vi "UpdateMotors.vi"(2 "Speed Fraction":dbl min=-1.0 max=1.0 step=0.01, 3 "Spin Fraction":dbl min=-1.0 max=1.0 step=0.001, 5 "Motor PWMs":T8) -> ()   [LabVIEW 2015]
uses:
  <vilib>/myRIO/Instrument Drivers/Onboard IO/PWM/typedefs/PWM Reference.ctl
  <vilib>/myRIO/Common/Instrument Driver Framework/Utilities/typedefs/myRIO Generic Hardware Reference.ctl
  <vilib>/myRIO/Common/Instrument Driver Framework/Utilities/typedefs/Hardware Version Enum.ctl
  <vilib>/myRIO/Common/Instrument Driver Framework/Utilities/typedefs/myRIO v1.0 Reference.ctl
  <vilib>/myRIO/Common/Instrument Driver Framework/Utilities/typedefs/Generic FPGA Reference.ctl
  <vilib>/myRIO/Common/Instrument Driver Framework/myRIO v1.0/PWM/typedefs/PWM Channels Enum.ctl
  <vilib>/myRIO/Instrument Drivers/Onboard IO/PWM/typedefs/PWM Configuration.ctl
  <vilib>/myRIO/Instrument Drivers/Onboard IO/PWM/vis/Set Duty Cycle and Frequency.vi
  <vilib>/Utility/error.llb/Error Cluster From Error Code.vi
  <vilib>/myRIO/Common/Instrument Driver Framework/myRIO v1.0/PWM/vis/myRIO v1.0 Write PWM.vi
  <vilib>/myRIO/Instrument Drivers/Onboard IO/PWM/PWM.lvlib
panel:
  out "Waveform Chart 2":dbl(graph)
  out "Waveform Chart":dbl(graph)
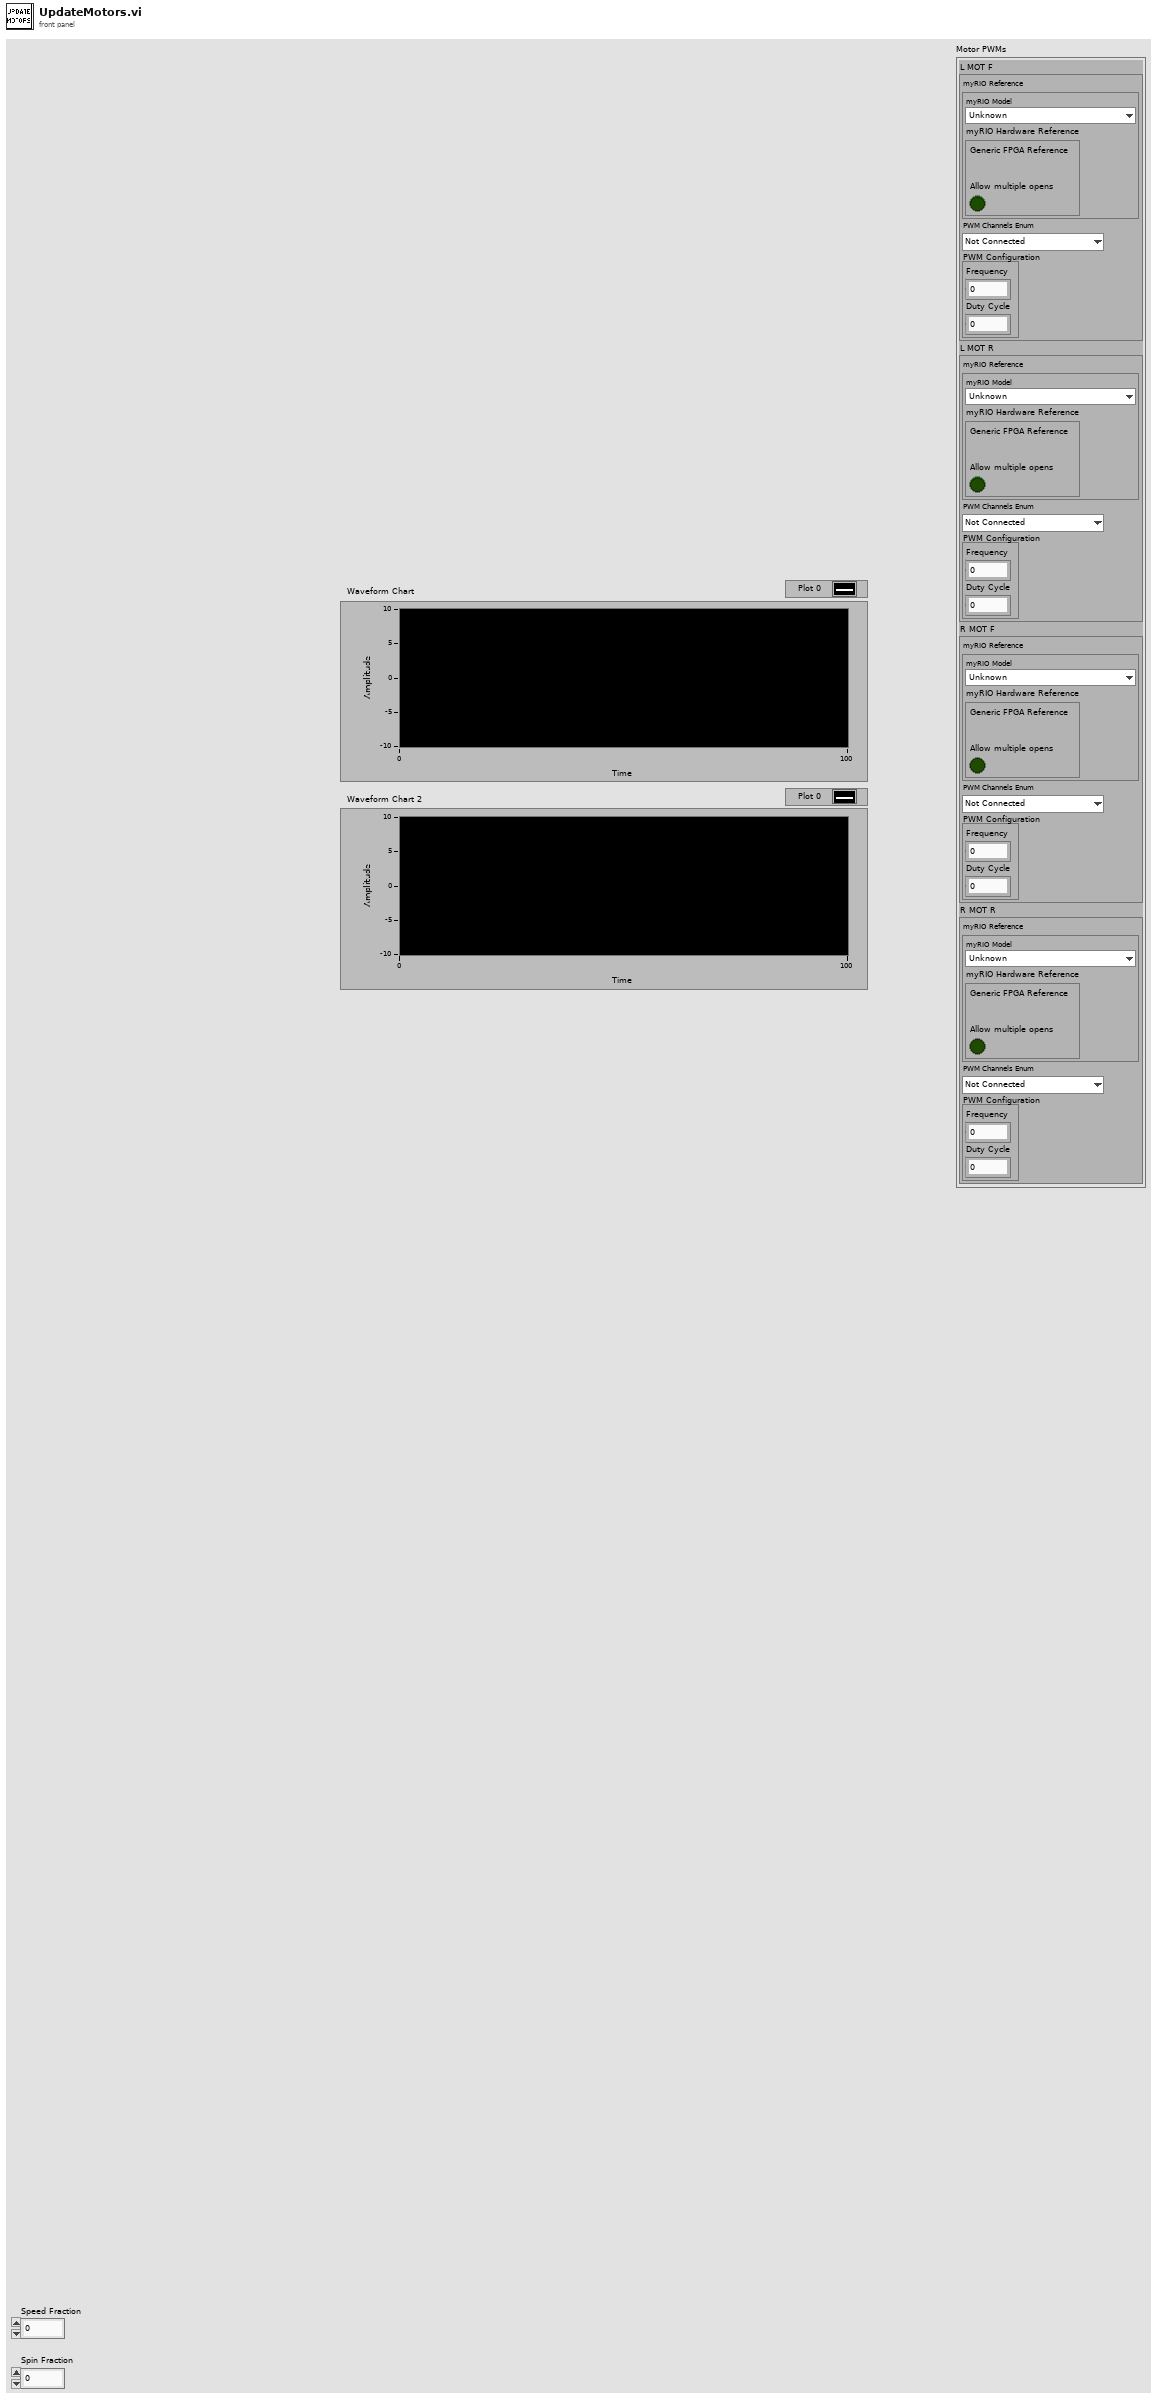
[diagram p1: front panel]
types:
  T1 = typedef "PWM.lvlib/PWM Reference.ctl" = cluster{"myRIO Reference":T2, "PWM Channels Enum":T6, "PWM Configuration":T7}
  T2 = typedef "myRIO Generic Hardware Reference.ctl" = cluster{"myRIO Model":T3, "myRIO Hardware Reference":T4}
  T3 = typedef "Hardware Version Enum.ctl" = enum16{"Unknown", "myRIO-1900", "myRIO-1950", "roboRIO"}
  T4 = typedef "myRIO v1.0 Reference.ctl" = cluster{"Generic FPGA Reference":T5, "Allow multiple opens":bool}
  T5 = typedef "Generic FPGA Reference.ctl" = refnum<k20>
  T6 = typedef "PWM Channels Enum.ctl" = enum16{"Not Connected", "C/PWM0", "C/PWM1", "A/PWM0", "A/PWM1", "A/PWM2", "B/PWM0", "B/PWM1", "B/PWM2", "PWM/PWM0", "PWM/PWM1", "PWM/PWM2", "PWM/PWM3", "PWM/PWM4", "PWM/PWM5", "PWM/PWM6", "PWM/PWM7", "PWM/PWM8", "PWM/PWM9"}
  T7 = typedef "PWM.lvlib/PWM Configuration.ctl" = cluster{"Frequency":dbl, "Duty Cycle":dbl}
  T8 = cluster{"L MOT F ":T1, "L MOT R":T1, "R MOT F":T1, "R MOT R":T1}
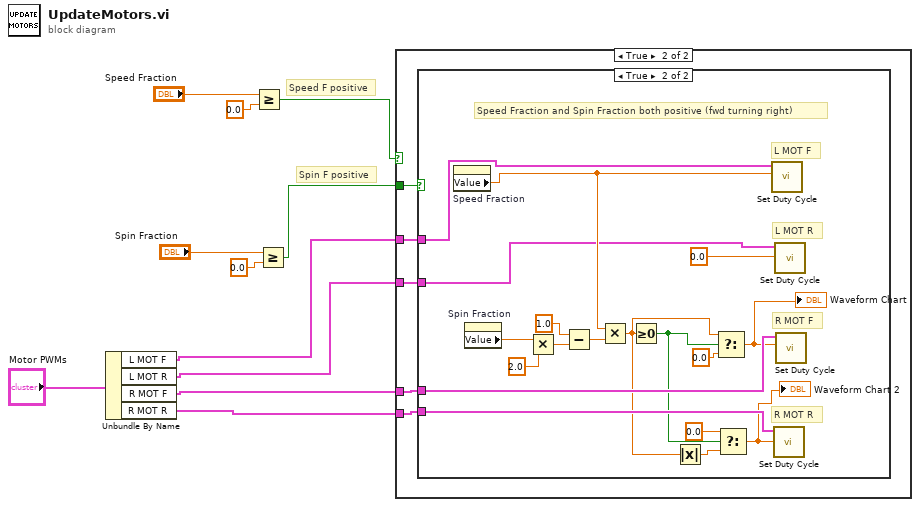
[diagram p0: block diagram]
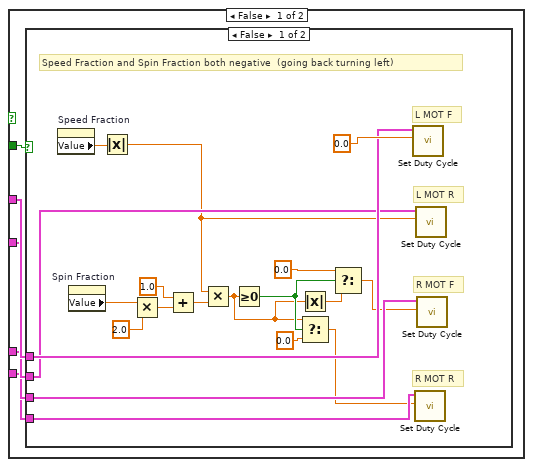
[diagram p2: hidden frame]
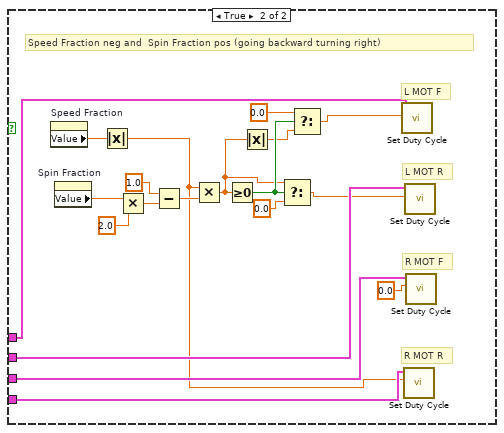
[diagram p3: hidden frame]
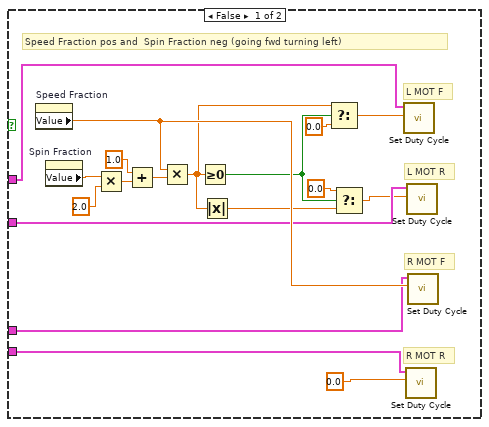
[diagram p4: hidden frame]
diagram:
  # "Spin F positive"
  # "Speed F positive"
  n1 = Unbundle By Name("Motor PWMs") -> ("L MOT F"=w5:T1, "L MOT R"=w4:T1, "R MOT F"=w3:T1, "R MOT R"=w2:T1)
  n2 = Greater Or Equal?(x="Speed Fraction", y=0.0) -> (x >= y?=w7:bool)
  n3 = Greater Or Equal?(x="Spin Fraction", y=0.0) -> (x >= y?=w6:bool)
  n4 = case shown="True" w7 {
    tunnel: w6 -> [w16 w59]
    tunnel: w5 -> [w15 w58]
    tunnel: w4 -> [w14 w57]
    tunnel: w3 -> [w13 w56]
    tunnel: w2 -> [w12 w55]
    frame False {
      n5 = case shown="False" w16 {
        tunnel: w15 -> [w29 w48]
        tunnel: w14 -> [w28 w47]
        tunnel: w13 -> [w27 w46]
        tunnel: w12 -> [w26 w45]
        frame False {
          # "Speed Fraction and Spin Fraction both negative  (going back turning left)"
          # "R MOT R"
          # "L MOT R"
          # "R MOT F"
          # "L MOT F"
          n6 = property on="Speed Fraction" class="DigNum (strict)"() -> ("Value"=w25:dbl)  [unwired: 2 in, 2 out]
          n7 = property on="Spin Fraction" class="DigNum (strict)"() -> ("Value"=w31:dbl)  [unwired: 2 in, 2 out]
          n8 = Absolute Value(x=w25) -> (abs(x)=w24:dbl)
          n9 = Multiply(x=w31, y=2.0) -> (x*y=w33:dbl)
          n10 = Add(x=1.0, y=w33) -> (x+y=w35:dbl)
          n11 = Multiply(x=w24, y=w35) -> (x*y=w19:dbl)
          n12 = Greater Or Equal To 0?(x=w19) -> (x >= 0?=w21:bool)
          n13 = Absolute Value(x=w19) -> (abs(x)=w18:dbl)
          n14 = Select(t=w19, s=w21, f=0.0) -> (s? t:f=w22:dbl)
          n15 = Select(t=0.0 ("Duty Cycle"), s=w21, f=w18) -> (s? t:f=w17:dbl)
          n16 = call <vilib>:"Set Duty Cycle.vi"("Duty Cycle"=0.0, "PWM Ref In"=w29) -> ()  [unwired: 7 in, 2 out]
          n17 = call <vilib>:"Set Duty Cycle.vi"("Duty Cycle"=w22, "PWM Ref In"=w26) -> ()  [unwired: 7 in, 2 out]
          n18 = call <vilib>:"Set Duty Cycle.vi"("Duty Cycle"=w24, "PWM Ref In"=w28) -> ()  [unwired: 7 in, 2 out]
          n19 = call <vilib>:"Set Duty Cycle.vi"("Duty Cycle"=w17, "PWM Ref In"=w27) -> ()  [unwired: 7 in, 2 out]
        }
        frame True {
          # "Speed Fraction neg and  Spin Fraction pos (going backward turning right)"
          # "R MOT R"
          # "L MOT R"
          # "R MOT F"
          # "L MOT F"
          n20 = property on="Speed Fraction" class="DigNum (strict)"() -> ("Value"=w44:dbl)  [unwired: 2 in, 2 out]
          n21 = property on="Spin Fraction" class="DigNum (strict)"() -> ("Value"=w54:dbl)  [unwired: 2 in, 2 out]
          n22 = Absolute Value(x=w44) -> (abs(x)=w43:dbl)
          n23 = Multiply(x=w54, y=2.0) -> (x*y=w52:dbl)
          n24 = Subtract(x=1.0, y=w52) -> (x-y=w50:dbl)
          n25 = Multiply(x=w43, y=w50) -> (x*y=w37:dbl)
          n26 = Greater Or Equal To 0?(x=w37) -> (x >= 0?=w39:bool)
          n27 = Absolute Value(x=w37) -> (abs(x)=w38:dbl)
          n28 = Select(t=w37, s=w39, f=0.0) -> (s? t:f=w42:dbl)
          n29 = Select(t=0.0 ("Duty Cycle"), s=w39, f=w38) -> (s? t:f=w36:dbl)
          n30 = call <vilib>:"Set Duty Cycle.vi"("Duty Cycle"=w36, "PWM Ref In"=w48) -> ()  [unwired: 7 in, 2 out]
          n31 = call <vilib>:"Set Duty Cycle.vi"("Duty Cycle"=w43, "PWM Ref In"=w45) -> ()  [unwired: 7 in, 2 out]
          n32 = call <vilib>:"Set Duty Cycle.vi"("Duty Cycle"=w42, "PWM Ref In"=w47) -> ()  [unwired: 7 in, 2 out]
          n33 = call <vilib>:"Set Duty Cycle.vi"("Duty Cycle"=0.0, "PWM Ref In"=w46) -> ()  [unwired: 7 in, 2 out]
        }
      }
    }
    frame True {
      n34 = case shown="True" w59 {
        tunnel: w58 -> [w70 w88]
        tunnel: w57 -> [w69 w87]
        tunnel: w56 -> [w68 w86]
        tunnel: w55 -> [w67 w85]
        frame False {
          # "Speed Fraction pos and  Spin Fraction neg (going fwd turning left)"
          # "R MOT R"
          # "L MOT R"
          # "R MOT F"
          # "L MOT F"
          n35 = property on="Speed Fraction" class="DigNum (strict)"() -> ("Value"=w71:dbl)  [unwired: 2 in, 2 out]
          n36 = property on="Spin Fraction" class="DigNum (strict)"() -> ("Value"=w77:dbl)  [unwired: 2 in, 2 out]
          n37 = Multiply(x=w77, y=2.0) -> (x*y=w75:dbl)
          n38 = Add(x=1.0, y=w75) -> (x+y=w73:dbl)
          n39 = Multiply(x=w71, y=w73) -> (x*y=w61:dbl)
          n40 = Greater Or Equal To 0?(x=w61) -> (x >= 0?=w63:bool)
          n41 = Absolute Value(x=w61) -> (abs(x)=w60:dbl)
          n42 = Select(t=w61, s=w63, f=0.0) -> (s? t:f=w66:dbl)
          n43 = Select(t=0.0, s=w63, f=w60) -> (s? t:f=w64:dbl)
          n44 = call <vilib>:"Set Duty Cycle.vi"("Duty Cycle"=w66, "PWM Ref In"=w70) -> ()  [unwired: 7 in, 2 out]
          n45 = call <vilib>:"Set Duty Cycle.vi"("Duty Cycle"=0.0, "PWM Ref In"=w67) -> ()  [unwired: 7 in, 2 out]
          n46 = call <vilib>:"Set Duty Cycle.vi"("Duty Cycle"=w64, "PWM Ref In"=w69) -> ()  [unwired: 7 in, 2 out]
          n47 = call <vilib>:"Set Duty Cycle.vi"("Duty Cycle"=w71, "PWM Ref In"=w68) -> ()  [unwired: 7 in, 2 out]
        }
        frame True {
          # "Speed Fraction and Spin Fraction both positive (fwd turning right)"
          # "R MOT R"
          # "L MOT R"
          # "R MOT F"
          # "L MOT F"
          n48 = property on="Speed Fraction" class="DigNum (strict)"() -> ("Value"=w90:dbl)  [unwired: 2 in, 2 out]
          n49 = property on="Spin Fraction" class="DigNum (strict)"() -> ("Value"=w95:dbl)  [unwired: 2 in, 2 out]
          n50 = Multiply(x=w95, y=2.0) -> (x*y=w93:dbl)
          n51 = Subtract(x=1.0, y=w93) -> (x-y=w91:dbl)
          n52 = Multiply(x=w90, y=w91) -> (x*y=w80:dbl)
          n53 = Greater Or Equal To 0?(x=w80) -> (x >= 0?=w83:bool)
          n54 = Absolute Value(x=w80) -> (abs(x)=w81:dbl)
          n55 = Select(t=w80, s=w83, f=0.0) -> (s? t:f=w79:dbl)
          "Waveform Chart" <- w79
          n56 = Select(t=0.0, s=w83, f=w81) -> (s? t:f=w78:dbl)
          "Waveform Chart 2" <- w78
          n57 = call <vilib>:"Set Duty Cycle.vi"("Duty Cycle"=w90, "PWM Ref In"=w88) -> ()  [unwired: 7 in, 2 out]
          n58 = call <vilib>:"Set Duty Cycle.vi"("Duty Cycle"=w78, "PWM Ref In"=w85) -> ()  [unwired: 7 in, 2 out]
          n59 = call <vilib>:"Set Duty Cycle.vi"("Duty Cycle"=0.0, "PWM Ref In"=w87) -> ()  [unwired: 7 in, 2 out]
          n60 = call <vilib>:"Set Duty Cycle.vi"("Duty Cycle"=w79, "PWM Ref In"=w86) -> ()  [unwired: 7 in, 2 out]
        }
      }
    }
  }
